vi "DecorationShow.vi"(8 "error in (no error)":errorcluster, 9 "Visible":bool, 10 "index":i32, 11 "VI_Ref":refnum<vi>) -> (0 "error out":errorcluster)   [LabVIEW 2025, in "UI_Library.lvlib" / "UI_Library.lvclass"]
doc: "Set Visible\\Unvisible a UI Decoration"
uses:
  UI_Library.lvclass
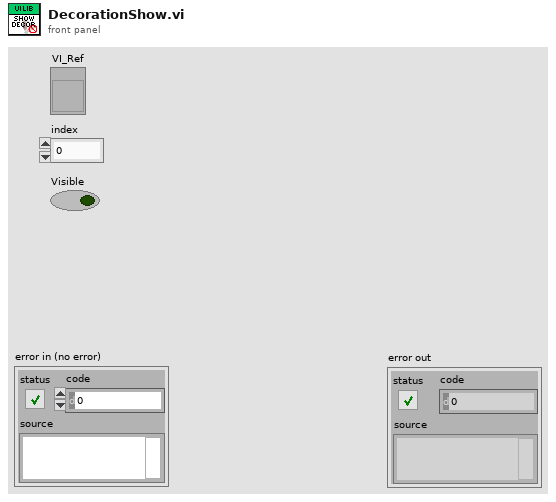
[diagram p1: front panel]
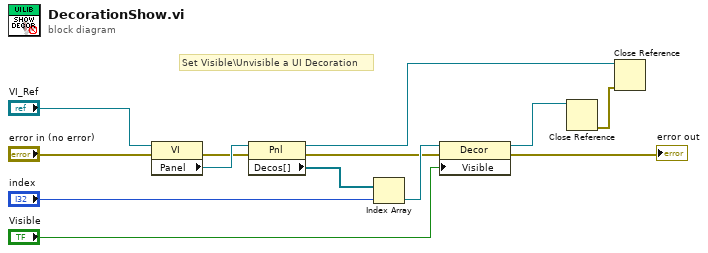
[diagram p0: block diagram]
diagram:
  # "Set Visible\\Unvisible a UI Decoration"
  n1 = property on="Property Node" class="VI"(reference="VI_Ref", error in="error in (no error)") -> (error out=w9:errorcluster, "Panel"=w13:refnum<vi>)  [unwired: 1 out]
  n2 = property on="Property Node" class="Pnl"(reference=w13, error in=w9) -> (reference out=w3:refnum<vi>, error out=w10:errorcluster, "Decos[]"=w12:refnum<vi>[])
  n3 = Index Array(array=w12, index="index") -> (element=w11:refnum<vi>)
  n4 = property on="Property Node" class="Decor"(reference=w11, error in=w10, "Visible"="Visible") -> (reference out=w8:refnum<vi>, error out=→"error out":errorcluster)
  n5 = Close Reference(reference=w8) -> (error out=w1:errorcluster)  [unwired: 1 in]
  n6 = Close Reference(reference=w3, error in (no error)=w1) -> ()  [unwired: 1 out]
